vi "Time series cursor boundary conditions.vi"(10 "XScale.Range":T2, 11 "Timeline Graph":T1) -> (2 "Maximum":dbl, 3 "Minimum":dbl)   [LabVIEW 2017, in "XGrapher.xctl"]
uses:
  XGrapher.xctl
  <vilib>/Utility/miscctls.llb/LVRangeTypeDef.ctl
  Typedefs/Xctrl-Timeline graph ref.ctl
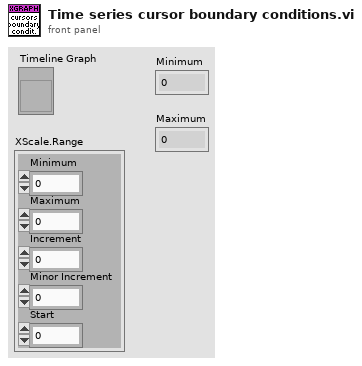
[diagram p1: front panel]
types:
  T1 = typedef "XGrapher.xctl/Xctrl-Timeline graph ref.ctl" = refnum<vi>
  T2 = typedef "LVRangeTypeDef.ctl" = cluster{"Minimum":dbl, "Maximum":dbl, "Increment":dbl, "Minor Increment":dbl, "Start":dbl}
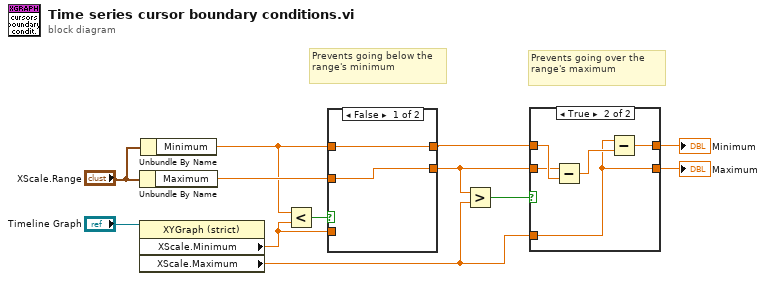
[diagram p0: block diagram]
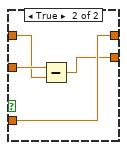
[diagram p3: hidden frame]
diagram:
  # "Prevents going over the range's maximum"
  # "Prevents going below the range's minimum"
  n1 = Unbundle By Name("XScale.Range") -> ("Maximum"=w12:dbl)
  n2 = property on="Property Node" class="XYGraph (strict)"(reference="Timeline Graph") -> ("XScale.Minimum"=w11:dbl, "XScale.Maximum"=w2:dbl)  [unwired: 1 in, 2 out]
  n3 = Unbundle By Name("XScale.Range") -> ("Minimum"=w8:dbl)
  n4 = Less?(x=w8, y=w11) -> (x < y?=w10:bool)
  n5 = case shown="False" w10 {
    tunnel: w11 -> [_ w18]
    tunnel: [w14 w18] -> w4
    tunnel: w8 -> [w14 w16]
    tunnel: w12 -> [w13 w17]
    tunnel: [w13 w15] -> w3
    frame False {
    }
    frame True {
      n6 = Subtract(x=w17, y=w16) -> (x-y=w15:dbl)
    }
  }
  n7 = Greater?(x=w3, y=w2) -> (0:w5:bool)
  n8 = case shown="True" w5 {
    tunnel: [w20 w22] -> w7
    tunnel: w4 -> [w20 w25]
    tunnel: w3 -> [w19 w24]
    tunnel: [w19 w21] -> w6
    tunnel: w2 -> [_ w21]
    frame False {
    }
    frame True {
      n9 = Subtract(x=w24, y=w25) -> (x-y=w23:dbl)
      n10 = Subtract(x=w21, y=w23) -> (x-y=w22:dbl)
    }
  }
  "Maximum" <- w6
  "Minimum" <- w7
